vi "Show config values.vi"(6 "wait for reply (T)":bool=TRUE, 8 "error in":errorcluster, 11 "Module ID":i32=-1) -> (0 "error out":errorcluster, 1 "timed out?":bool, 2 "params":T1, 3 "Module ID out":i32)   [LabVIEW 2021, in "Communication.lvlib"]
doc: "This event show the values read from config file\n\n_____\nCreated using DQMH Framework: Event Scripter 7.1.2.1547."
uses:
  Communication.lvlib
  Show config values Argument--cluster.ctl
  Show config values (Reply Payload)--cluster.ctl
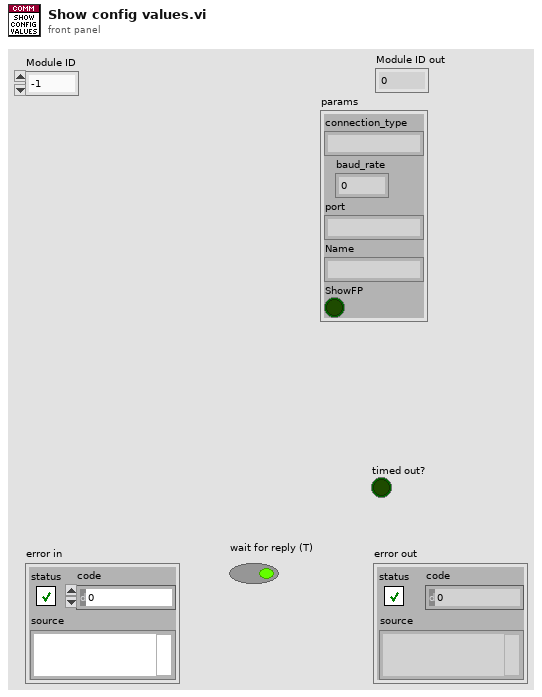
[diagram p1: front panel]
types:
  T1 = cluster{"connection_type":string, "baud_rate":i32, "port":string, "Name":string, "ShowFP":bool}
  T2 = typedef "Communication.lvlib/Show config values Argument--cluster.ctl" = cluster{"Module ID":i32, "Wait Notifier":refnum<notifier>, "wait for reply":bool}
  T3 = typedef "Communication.lvlib/Request Events--cluster.ctl" = cluster{"Stop Module":refnum<user-event>, "Show Panel":refnum<user-event>, "Hide Panel":refnum<user-event>, "Show Diagram":refnum<user-event>, "Get Module Execution Status":refnum<user-event>, "Show config values":refnum<user-event>}
  T4 = typedef "Communication.lvlib/Show config values (Reply Payload)--cluster.ctl" = cluster{"Module ID":i32, "Comm":cluster{"Path":path}, "error":errorcluster, "params":cluster{"connection_type":string, "baud_rate":i32, "port":string, "Name":string, "ShowFP":bool}}
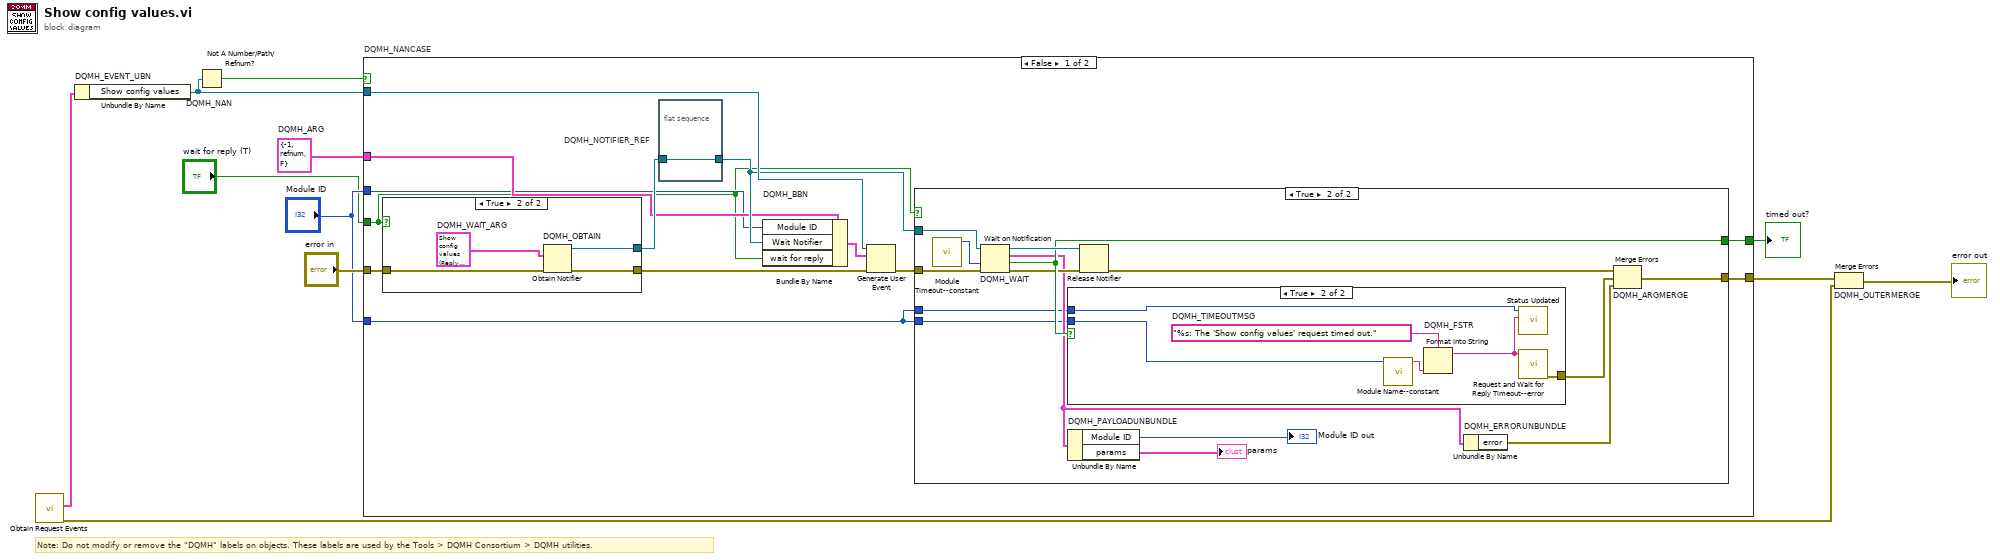
[diagram p0: block diagram]
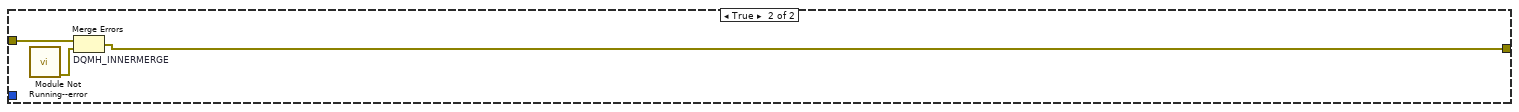
[diagram p5: hidden frame]
diagram:
  w5 = T2 {"Module ID"=-1, "Wait Notifier"=refnum, "wait for reply"=FALSE}  # DQMH_ARG
  # "Note: Do not modify or remove the \"DQMH\" labels on objects. These labels are used by the Tools > DQMH Consortium > DQMH utilities."
  n1 = call "Obtain Request Events.vi"() -> ("error out"=w2:errorcluster, "Communication Request Events"=w1:T3)  [unwired: 10 in]
  n2 = Unbundle By Name "DQMH_EVENT_UBN"(w1) -> ("Show config values"=w9:refnum<user-event>)
  n3 = Not A Number/Path/Refnum? "DQMH_NAN"(number/path/refnum=w9) -> (NaN/Path/Refnum?=w8:bool)
  n4 = case "DQMH_NANCASE" shown="False" w8 {
    tunnel: "error in" -> [w24 w55]
    tunnel: w9 -> [w22 _]
    tunnel: [w19 w54] -> w6
    tunnel: [w20 _] -> w7
    tunnel: w5 -> [w15 _]
    tunnel: "Module ID" -> [w14 _]
    tunnel: "Module ID" -> [w13 _]
    tunnel: "wait for reply (T)" -> [w12 _]
    frame False {
      n5 = case shown="True" w12 {
        tunnel: w24 -> [w48 w52]
        tunnel: [w48 w51] -> w21
        tunnel: [_ w49] -> w17
        frame False {
        }
        frame True {
          w50 = T4 {"Module ID"=-1, "Comm"={"Path"=path ""}, "error"={"status"=FALSE, "code"=0, "source"=""}, "params"={"connection_type"="", "baud_rate"=0, "port"="", "Name"="", "ShowFP"=FALSE}}  # DQMH_WAIT_ARG
          n6 = Obtain Notifier "DQMH_OBTAIN"(notification data type=w50, error in (no error)=w52) -> (notifier out=w49:refnum<notifier>, error out=w51:errorcluster)  [unwired: 2 in, 1 out]
        }
      }
      n7 = flat-sequence "DQMH_NOTIFIER_REF" {
        tunnel: w17 -> [w25]
        tunnel: [w25] -> w16
        frame #0 {
        }
      }
      n8 = Bundle By Name "DQMH_BBN"(cluster=w15, "Module ID"=w14, "Wait Notifier"=w16, "wait for reply"=w12) -> (w18:T2)
      n9 = Generate User Event(user event=w22, event data cluster=w18, error in=w21) -> (error out=w23:errorcluster)  [unwired: 1 in, 1 out]
      n10 = case shown="True" w12 {
        tunnel: w23 -> [w26 w41]
        tunnel: w16 -> [_ w40]
        tunnel: [_ w38] -> w20
        tunnel: [w26 w37] -> w19
        tunnel: w13 -> [_ w30]
        tunnel: w13 -> [_ w29]
        frame False {
        }
        frame True {
          n11 = call "Module Timeout--constant.vi"() -> ("Module Timeout"=w31:i32)  [unwired: 11 in]
          n12 = Wait on Notification "DQMH_WAIT"(notifier=w40, timeout in ms (-1)=w31, error in (no error)=w41) -> (notifier out=w39:refnum<notifier>, notification=w32:T4, timed out?=w38:bool, error out=w36:errorcluster)  [unwired: 1 in]
          n13 = case shown="True" w38 {
            tunnel: [_ w45] -> w33
            tunnel: w30 -> [_ w43]
            tunnel: w29 -> [_ w42]
            frame False {
            }
            frame True {
              w47 = "%s: The 'Show config values' request timed out."  # DQMH_TIMEOUTMSG
              n14 = call "Module Name--constant.vi"("Module ID"=w42) -> ("Module Name"=w44:string)  [unwired: 10 in]
              n15 = Format Into String "DQMH_FSTR"(format string=w47, w44) -> (resulting string=w46:string)  [unwired: 2 in, 1 out]
              n16 = call "Status Updated.vi"("Status"=w46, "Module ID"=w43) -> ()  [unwired: 9 in, 1 out]
              n17 = call "Request and Wait for Reply Timeout--error.vi"("Error Message"=w46) -> ("error out"=w45:errorcluster)  [unwired: 10 in]
            }
          }
          n18 = Unbundle By Name "DQMH_PAYLOADUNBUNDLE"(w32) -> ("Module ID"=→"Module ID out":i32, "params"=→"params":T1)
          n19 = Release Notifier(notifier=w39, error in (no error)=w36) -> (error out=w35:errorcluster)  [unwired: 1 in, 2 out]
          n20 = Unbundle By Name "DQMH_ERRORUNBUNDLE"(w32) -> ("error"=w34:errorcluster)
          n21 = Merge Errors "DQMH_ARGMERGE"(w35, w33, w34) -> (w37:errorcluster)
        }
      }
    }
    frame True {
      n22 = call "Module Not Running--error.vi"() -> ("error out"=w53:errorcluster)  [unwired: 11 in]
      n23 = Merge Errors "DQMH_INNERMERGE"(w55, w53) -> (w54:errorcluster)
    }
  }
  "timed out?" <- w7
  n24 = Merge Errors "DQMH_OUTERMERGE"(w6, w2) -> (→"error out":errorcluster)
